vi "New Verify.vi"   [LabVIEW 2020, in "Caraya.Extension.lvlib"]
uses:
  Approval Tests/Options/Options.lvclass/Options.ctl
  Approval Tests/Naming Data/Naming Data.lvclass/Naming Data.ctl
  Approval Tests/Options/Options.lvclass
  Approval Tests/Scrubber/Scrubber.lvclass
  Approval Tests/Namer/Namer.lvclass
  Approval Tests/Naming Data/Naming Data.lvclass
  Approval Tests/Reporter/Reporter.lvclass
  Approval Tests/Text Comparator/Text Comparator.lvclass
  Caraya.Extension.lvlib
  d4b99bd2-5c08-4417-935f-9c9e21584bf9.vi
  <vilib>/addons/_JKI Toolkits/Caraya/classes/Test/Test.lvclass
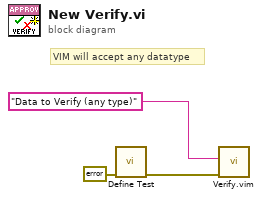
[diagram p0: block diagram]
diagram:
  # "VIM will accept any datatype"
  n1 = call <vilib>:"Define Test.vi"("error in (no error)"=errorcluster {"status"=FALSE, "code"=0, "source"=""}) -> ("error out"=w2:errorcluster)  [unwired: 9 in, 1 out]
  n2 = call "Verify.vim"("error in"=w2, "Test Data"="Data to Verify (any type)") -> ()  [unwired: 8 in, 2 out]
